vi "Init.vi"(8 "error in (no error)":errorcluster, 11 "Local Error Manager in":refnum<class "Local Error Manager.lvclass">) -> (0 "error out":errorcluster, 3 "Local Error Manager out":refnum<class "Local Error Manager.lvclass">)   [LabVIEW 2026, in "TALOS.lvlib" / "Error Manager.lvlib" / "Local Error Manager.lvclass"]
uses:
  Local Error Manager.lvclass
  C:/LabVIEW Code/TALOS/talos/Internal uServices/System uServices/Error Manager/Error Manager.lvclass
  Error Manager.lvclass/Error Manager.ctl
  Ancestor/Ancestor/Ancestor.lvclass/Ancestor.ctl
  Local Error Manager.lvclass/Local Error Manager.ctl
  Write Distributed flag.vi
  Write Distributed Error Manager Started flag.vi
  Write Distributed Mngr Status.vi
  Support VIs/Generate Error.vi
  FGV/Error Memory/Get Error Description.vi
  Support VIs/Get PC name.vi
  Ancestor/Ancestor/Read ID.vi
  Support VIs/Get Class Name.vi
  <vilib>/Utility/error.llb/Clear Errors.vi
  FGV/Error Memory/Error Memory Core.vi
  <vilib>/AdvancedString/Delimited String to 1D String Array.vi
  <vilib>/AdvancedString/Delimited String to 1D String Array (string).vi
  Support VIs/Circus Root Path.vi
  FGV/Error Memory/Error Crt Lvl checker.vi
  FGV/Error Memory/Error Memory Core.vi/40c8088d-b597-4017-91af-faa98e00292e.vi
  FGV/Error Memory/Error Memory Core.vi/d4a3ab98-063c-4e44-b43d-fbdcfe6c2be2.vi
  Support VIs/Global Memory.vi
  <vilib>/Utility/LVClass/Get LV Class Name.vi
  Support VIs/Is in Packed Library.vi
  Support VIs/TALOS Root path.vi
  Support VIs/Read CSV worksheet.vi
  Support VIs/Global Constants.vi
  <vilib>/Utility/error.llb/General Error Handler.vi
  <vilib>/Utility/config.llb/Open Config Data.vi
  <vilib>/Utility/config.llb/Get Section Names.vi
  <vilib>/Utility/config.llb/Get Key Names.vi
  <vilib>/Utility/config.llb/Read Key.vi
  <vilib>/Utility/config.llb/Read Key (String).vi
  <vilib>/Utility/config.llb/Close Config Data.vi
  <vilib>/Utility/error.llb/Search and Replace Pattern.vi
  <vilib>/Utility/error.llb/Search and Replace Pattern (string).vi
  Ancestor/Ancestor/Ancestor.lvclass
  <vilib>/Comparison/Equal/Equal Functor/Equal Functor.lvclass
  Error Manager.lvclass
  TALOS.lvlib
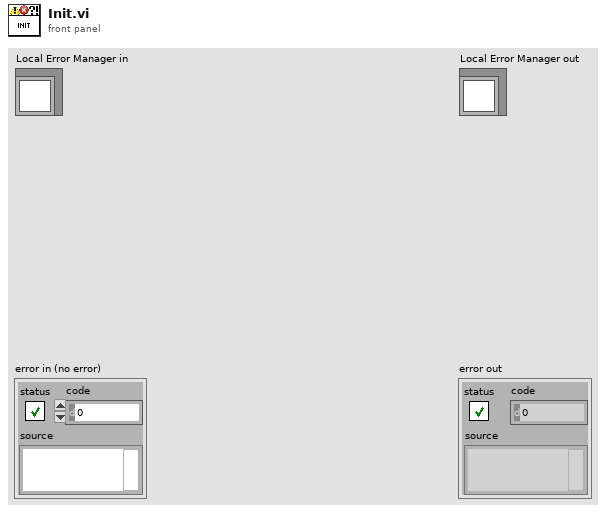
[diagram p1: front panel]
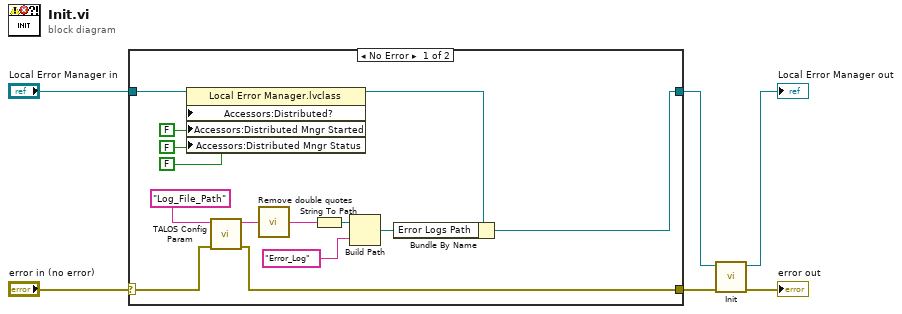
[diagram p0: block diagram]
diagram:
  n1 = case shown="No Error" "error in (no error)" {
    selector: "error in (no error)" -> [w15 w22]
    tunnel: [w8 w22] -> w4
    tunnel: [w9 w21] -> w2
    tunnel: "Local Error Manager in" -> [w14 w21]
    frame No Error {
      n2 = property class="Local Error Manager.lvclass"(reference=w14, "Accessors:Distributed?"=FALSE ("Update listbox"), "Accessors:Distributed Mngr Started"=FALSE ("Global Mgr Started"), "Accessors:Distributed Mngr Status"=FALSE ("Distributed Mngr Status")) -> (reference out=w12:refnum<class "Local Error Manager.lvclass">)  [unwired: 1 in, 1 out]
      n3 = call "TALOS Config Param.vi"("error in (no error)"=w15, "Parameter Name"="Log_File_Path") -> ("error out"=w8:errorcluster, "Output"=w17:string)  [unwired: 8 in]
      n4 = call "Remove double quotes.vi"("Input string"=w17) -> ("Output string"=w18:string)  [unwired: 4 in]
      n5 = String To Path(string=w18) -> (path=w19:path)
      n6 = Build Path(base path=w19, name or relative path="Error_Log") -> (appended path=w13:path)
      n7 = Bundle By Name(cluster=w12, "Error Logs Path"=w13) -> (w9:refnum<class "Local Error Manager.lvclass">)
    }
    frame Error {
    }
  }
  n8 = call-parent "Init.vi"("error in (no error)"=w4, "uService Template in"=w2) -> ("error out"=→"error out":errorcluster, "uService Template out"=→"Local Error Manager out":refnum<class "Local Error Manager.lvclass">)  [unwired: 8 in]
